vi "子VI-查看某框-不显示界面.vi"(0 "框号":dbl format="%#_13g", 1 "框组":T3(array[cluster]), 2 "计入缺陷的Z值阈值":i32 caption="值", 3 "临界Z值":i32, 4 "计入缺陷的面积阈值":i32, 5 "临界面积百分比值":dbl, 6 "图像Y向分辨率（mm/像素）":dbl, 7 "缺陷灰度阈值":dbl caption="值", 8 "?":T2(plugin-control), 9 "部位信息":string[](array[string])=["", "34.500000", "32.500000", "1121", "34", "54.955926", "分层类", "不合格", ""], 10 "判定为筋条的长宽比阈值":i32, 11 "图像X向分辨率（mm/像素）":dbl) -> (20 "全部检测结果":string[][](table))   [LabVIEW 2018]
uses:
  <vilib>/vision/NI_Vision_Development_Module.lvlib
panel:
  out "中心Y":dbl
  out "中心X":dbl
  in  "Tab Control":T1
  out "Threshold Image":T2(plugin-control)
  out "分层缺陷个数":i32
  out "合格？ 弥散类":string="fencengThreshold"
  out "合格？分层类":string="fencengThreshold"
  out "面积 (pixels)":i32
  in  "格式字符串 2":string="%f"
  in  "分隔符（'\\'代码显示）":string="\t"
  out "分层测量结果":i16[][](array[numeric])
  # "所选区域信息"
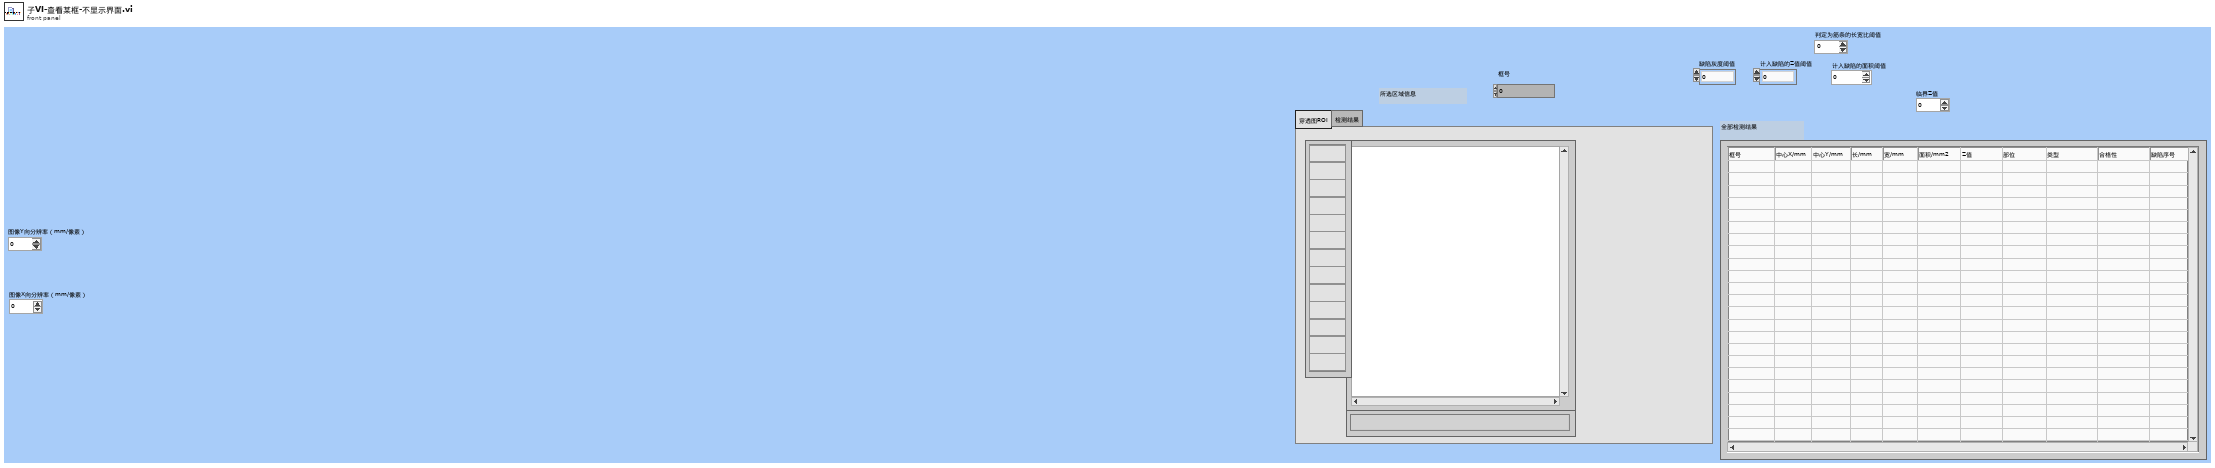
[diagram p1: front panel]
types:
  T1 = typedef "控件2.ctl" = enum32{"穿透图ROI", "检测结果"}
  T2 = typedef "IMAQ Image.ctl" = refnum<image>
  T3 = cluster{"Global Rectangle":i32[], "Contours":cluster{"Contour Type":u32, "ROI Type":u32, "Points":i32[]}[]}[]
  T4 = typedef "Image Type" = u32
  T5 = cluster{"Global Rectangle":i32[], "Contours":cluster{"Contour Type":u32, "ROI Type":u32, "Points":i32[]}[]}
  T6 = cluster{"Desired Font (Application)":enum16{"User-specified Font", "Application Font", "System Font", "Dialog Font"}, "[User-specified Font]":cluster{"Font Name":string, "Size":i16, "Strikeout?":bool, "Italic?":bool, "Underline?":bool, "Outline?":bool, "Shadow?":bool, "Bold?":bool, "Rotation Angle":dbl}, "Horizontal Alignment":i16, "Vertical Alignment":i16}
  T7 = cluster{"histogram":u32[], "Minimal Value":sgl, "Maximal Value":sgl, "Starting Value":sgl, "Interval Width":sgl, "Mean Value":sgl, "Standard  Variation":sgl, "Area (pixels)":i32}
  T8 = typedef "Particle Parameters" = i32
  T9 = cluster{"Area":dbl, "Number of Holes":dbl, "Bounding Rect":cluster{"Left":dbl, "Top":dbl, "Right":dbl, "Bottom":dbl}, "Center of Mass":cluster{"X":dbl, "Y":dbl}, "Orientation":dbl, "Dimensions":cluster{"Width":dbl, "Height":dbl}}[]
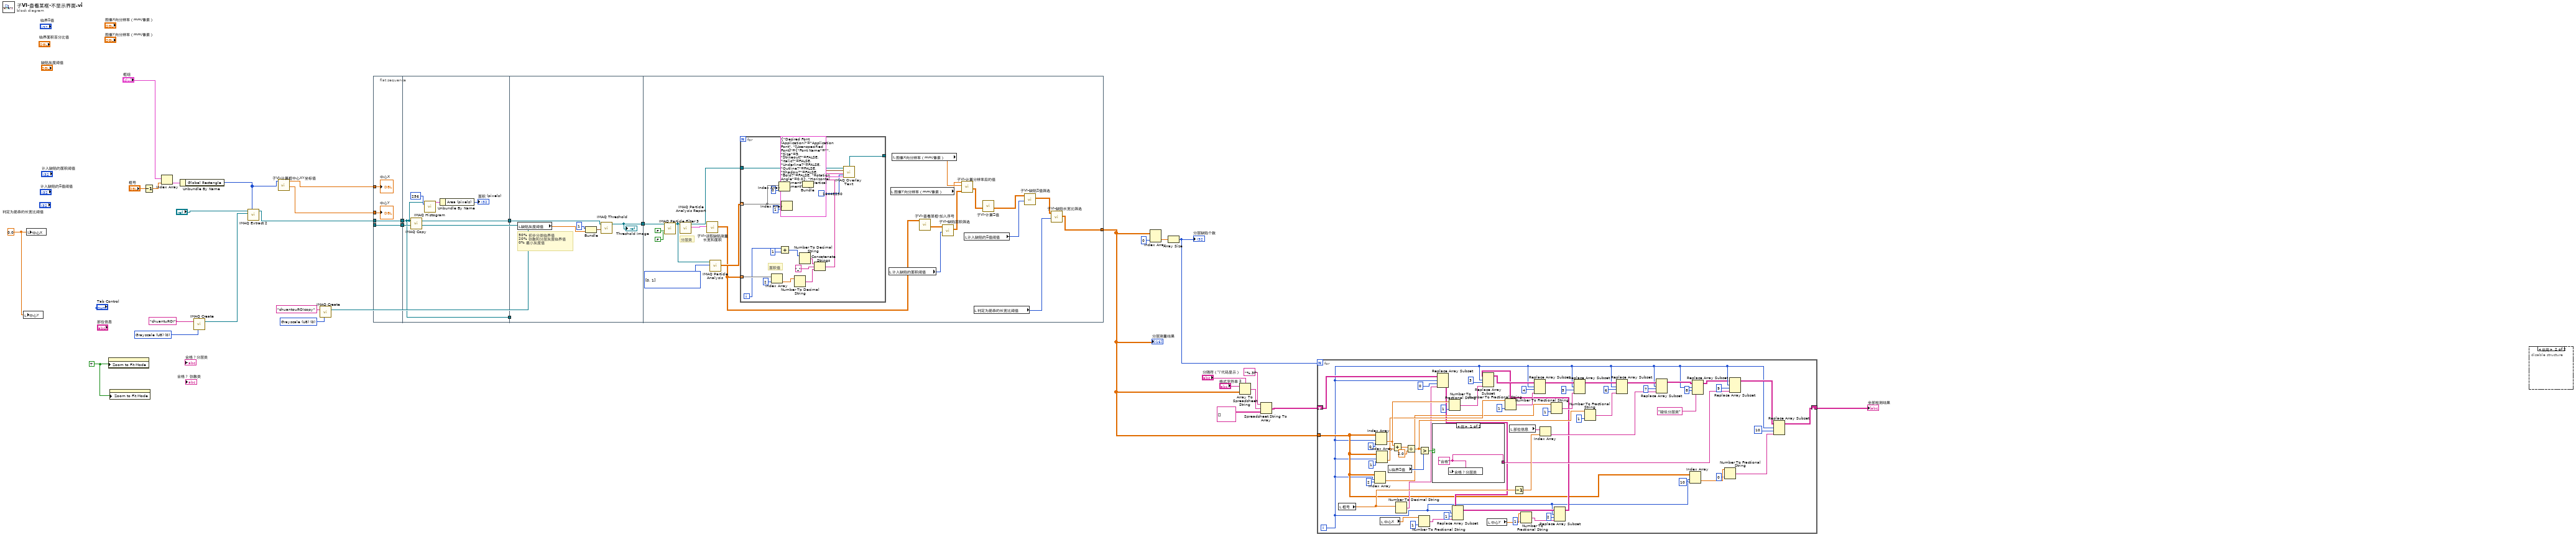
[diagram p0: block diagram]
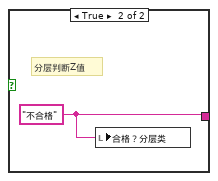
[diagram p2: hidden frame]
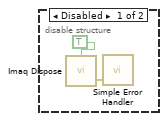
[diagram p3: hidden frame]
diagram:
  w4 = 0.0 ("中心X")
  w8 = T4 0 items=["Grayscale (U8)", "Grayscale (I16)", "Grayscale (SGL)", "Complex (CSG)", "RGB (U32)", "HSL (U32)", "RGB (U64)", "Grayscale (U16)"] ("Image Type")
  w13 = TRUE ("Zoom to Fit Mode")
  w28 = T4 0 items=["Grayscale (U8)", "Grayscale (I16)", "Grayscale (SGL)", "Complex (CSG)", "RGB (U32)", "HSL (U32)", "RGB (U64)", "Grayscale (U16)"] ("Image Type")
  n1 = local write "中心Y"(w4) -> ()
  n2 = local write "中心X"(w4) -> ()
  n3 = property class="ImageControl"("Zoom to Fit Mode"=w13) -> ()  [unwired: 2 in, 2 out]
  n4 = property class="ImageControl"("Zoom to Fit Mode"=w13) -> ()  [unwired: 2 in, 2 out]
  n5 = Decrement(x="框号") -> (x-1=w30:dbl)
  n6 = Index Array(array="框组", index=w30) -> (element=w31:T5)
  n7 = Unbundle By Name(w31) -> ("Global Rectangle"=w7:i32[])
  n8 = call "IMAQ Create"("Image Name"="chuantuROI", "Image Type"=w28) -> ("New Image"=w27:T2)  [unwired: 3 in, 1 out]
  n9 = call "IMAQ Extract 2"("Optional Rectangle"=w7, "Image Dst"=w27, "Image Src"="?") -> ("Image Dst Out"=w1:T2)  [unwired: 7 in, 1 out]
  n10 = call "子VI-计算框中心XY坐标值.vi"("Global Rectangle"=w7) -> ("中心Y"=w5:dbl, "中心X"=w6:dbl)  [unwired: 9 in]
  n11 = call "IMAQ Create"("Image Name"="chuantouROIcopy", "Image Type"=w8) -> ("New Image"=w11:T2)  [unwired: 3 in, 1 out]
  n12 = flat-sequence {
    tunnel: w1 -> [w37]
    tunnel: [w37] -> w14
    tunnel: w11 -> [w36]
    tunnel: [w36] -> w10
    tunnel: w6 -> [w35]
    tunnel: w5 -> [w34]
    tunnel: [w40] -> w15
    tunnel: w14 -> [w40]
    tunnel: [w39] -> w12
    tunnel: w10 -> [w38]
    tunnel: [w48] -> w24
    tunnel: w15 -> [_]
    tunnel: w12 -> [w47]
    tunnel: [w60] -> w17
    tunnel: w24 -> [w66]
    frame #0 {
      "中心X" <- w35
      "中心Y" <- w34
    }
    frame #1 {
      n13 = call "IMAQ Copy"("Image Dst"=w38, "Image Src"=w40) -> ("Image Dst Out"=w39:T2)  [unwired: 4 in, 1 out]
      n14 = call "IMAQ Histogram"("Number of Classes"=256, "Image"=w40) -> ("Histogram Report"=w42:T7)  [unwired: 8 in, 1 out]
      n15 = Unbundle By Name(w42) -> ("Area (pixels)"=→"面积 (pixels)":i32)
    }
    frame #2 {
      # "50% 初步分类临界值\n20% 弥散和分层灰度临界值\n0% 最小灰度值"
      n16 = local read "缺陷灰度阈值"() -> (w45:dbl)
      n17 = Bundle(1, "缺陷灰度阈值"=w45) -> (w44:cluster{i32, "缺陷灰度阈值":dbl})  [unwired: 1 in]
      n18 = call "IMAQ Threshold"("Range"=w44, "Image Src"=w47) -> ("Image Dst Out"=w48:T2)  [unwired: 4 in, 5 out]
      "Threshold Image" <- w48
    }
    frame #3 {
      w54 = T8[] [0, 1] items=["Center of Mass X", "Center of Mass Y", "First Pixel X", "First Pixel Y", "Bounding Rect Left", "Bounding Rect Top", "Bounding Rect Right", "Bounding Rect Bottom", "Max Feret Diameter Start X", "Max Feret Diameter Start Y", "Max Feret Diameter End X", "Max Feret Diameter End Y", "Max Horiz. Segment Length Left", "Max Horiz. Segment Length Right", "Max Horiz. Segment Length Row", "-", "Bounding Rect Width", "Bounding Rect Height", "Bounding Rect Diagonal", "Perimeter", "Convex Hull Perimeter", "Holes' Perimeter", "Max Feret Diameter", "Equivalent Ellipse Major Axis", "Equivalent Ellipse Minor Axis", "Equivalent Ellipse Minor Axis (Feret)", "Equivalent Rect Long Side", "Equivalent Rect Short Side", "Equivalent Rect Diagonal", "Equivalent Rect Short Side (Feret)", "Average Horiz. Segment Length", "Average Vert. Segment Length", "Hydraulic Radius", "Waddel Disk Diameter", "-", "Area", "Holes' Area", "Particle & Holes' Area", "Convex Hull Area", "Image Area", "-", "Number of Holes", "Number of Horiz. Segments", "Number of Vert. Segments", "-", "Orientation", "Max Feret Diameter Orientation", "-", "% Area/Image Area", "% Area/(Particle & Holes' Area)", "Ratio of Equivalent Ellipse Axes", "Ratio of Equivalent Rect Sides", "-", "Elongation Factor", "Compactness Factor", "Heywood Circularity Factor", "Type Factor", "-", "Sum X", "Sum Y", "Sum XX", "Sum XY", "Sum YY", "Sum XXX", "Sum XXY", "Sum XYY", "Sum YYY", "-", "Moment of Inertia XX", "Moment of Inertia XY", "Moment of Inertia YY", "Moment of Inertia XXX", "Moment of Inertia XXY", "Moment of Inertia XYY", "Moment of Inertia YYY", "Norm. Moment of Inertia XX", "Norm. Moment of Inertia XY", "Norm. Moment of Inertia YY", "Norm. Moment of Inertia XXX", "Norm. Moment of Inertia XXY", "Norm. Moment of Inertia XYY", "Norm. Moment of Inertia YYY", "Hu Moment 1", "Hu Moment 2", "Hu Moment 3", "Hu Moment 4", "Hu Moment 5", "Hu Moment 6", "Hu Moment 7"] ("Pixel Measurements")
      # "分层类"
      n19 = call "IMAQ Particle Filter 3"("Image Src"=w66, "Keep/Remove Particles (F)"=FALSE, "Reject Border? (F)"=FALSE) -> ("Image Dst Out"=w53:T2)  [unwired: 10 in, 2 out]
      n20 = call "IMAQ Particle Analysis Report"("Image"=w53) -> ("Particle Reports (Pixels)"=w65:T9, "Image Out (duplicate)"=w51:T2)  [unwired: 5 in, 4 out]
      n21 = call "子VI-读取缺陷测量长宽和面积.vi"("Particle Reports (Pixels)"=w65) -> ("测量结果"=w50:dbl[][])  [unwired: 10 in]
      n22 = call "IMAQ Particle Analysis"("Pixel Measurements"=w54, "Image"=w53) -> ("Particle Measurements (Pixels)"=w52:dbl[][])  [unwired: 4 in, 5 out]
      n23 = for {
        tunnel: [w80] -> _
        tunnel: w51 -> [w88]
        tunnel: w52 -> [w85] mode=indexing
        tunnel: w50 -> [w76] mode=indexing
        i -> [w71]
        # "面积值"
        n24 = Index Array(array=w76, index=2 ("索引")) -> (element=w83:dbl)
        n25 = Index Array(array=w85, index=0 ("索引")) -> (element=w79:dbl)
        n26 = Add(x=w71, y=1) -> (x+y=w69:i32)
        n27 = Index Array(array=w85, index=1 ("索引")) -> (element=w78:dbl)
        n28 = Number To Decimal String(number=w83) -> (decimal integer string=w73:string)  [unwired: 1 in]
        n29 = Number To Decimal String(number=w69) -> (decimal integer string=w75:string)  [unwired: 1 in]
        n30 = Bundle("Numeric"=w79, "Numeric"=w78) -> (w77:cluster{"Numeric":dbl, "Numeric":dbl})  [unwired: 1 in]
        n31 = Concatenate Strings(w75, "_" ("字符串"), w73) -> (w74:string)
        n32 = call "IMAQ Overlay Text"("Text Color (black)"=u32 16448250, "Font, Size & Style"=T6 {"Desired Font (Application)"=enum."Application Font", "[User-specified Font]"={"Font Name"="", "Size"=9, "Strikeout?"=FALSE, "Italic?"=FALSE, "Underline?"=FALSE, "Outline?"=FALSE, "Shadow?"=FALSE, "Bold?"=FALSE, "Rotation Angle"=0.0}, "Horizontal Alignment"=0, "Vertical Alignment"=0}, "String"=w74, "Origin"=w77, "Image"=w88) -> ("Image Out"=w80:T2)  [unwired: 5 in, 1 out]
      }
      n33 = local read "计入缺陷的面积阈值"() -> (w64:i32)
      n34 = local read "图像Y向分辨率（mm/像素）"() -> (w55:dbl)
      n35 = local read "图像X向分辨率（mm/像素）"() -> (w56:dbl)
      n36 = call "子VI-查看某框-加入序号.vi"("测量结果"=w50) -> ("测量结果 3"=w49:dbl[][])  [unwired: 9 in]
      n37 = call "子VI-缺陷面积筛选.vi"("计入分层缺陷的面积阈值"=w64, "分层测量结果"=w49) -> ("初始化的数组"=w58:dbl[][])  [unwired: 8 in, 1 out]
      n38 = call "子VI-计算分辨率后的值.vi"("测量结果"=w58, "图像X向分辨率（mm/像素）"=w56, "图像Y向分辨率（mm/像素）"=w55) -> ("初始化的数组"=w57:dbl[][])  [unwired: 7 in]
      n39 = local read "计入缺陷的Z值阈值"() -> (w63:i32)
      n40 = local read "判定为筋条的长宽比阈值"() -> (w59:i32)
      n41 = call "子VI-计算Z值.vi"("分层测量结果"=w57) -> ("初始化的数组"=w62:dbl[][])  [unwired: 9 in]
      n42 = call "子VI-缺陷Z值筛选.vi"("计入缺陷的Z值阈值"=w63, "分层测量结果"=w62) -> ("初始化的数组"=w61:dbl[][])  [unwired: 8 in, 1 out]
      n43 = call "子VI-缺陷长宽比筛选.vi"("判定为筋条的长宽比阈值"=w59, "分层测量结果"=w61) -> ("初始化的数组"=w60:dbl[][])  [unwired: 9 in]
    }
  }
  n44 = Index Array(array=w17, index (col)=0 ("禁用的索引 (列)")) -> (element=w26:dbl[])  [unwired: 1 in]
  n45 = Array Size(array=w26) -> (size(s)=w23:i32)
  "分层缺陷个数" <- w23
  n46 = Array To Spreadsheet String(delimiter (Tab)="分隔符（'\\'代码显示）", array=w17, 3:"格式字符串 2") -> (spreadsheet string=w20:string)
  n47 = Spreadsheet String To Array(format string="%.3f", spreadsheet string=w20, array type (2D Dbl)=string[][] [] ("Array")) -> (array=w16:string[][])  [unwired: 1 in]
  n48 = for {
    N: w23 -> [_]
    tunnel: w17 -> [w95]
    shift-right: [w99] -> w3
    shift-left: w16 -> [w133]
    i -> [w92]
    n49 = local read "框号"() -> (w140:dbl)
    n50 = Index Array(array=w95, index (row)=w92, index (col)=2 ("索引 (列)")) -> (element=w118:dbl)
    n51 = Index Array(array=w95, index (row)=w92, index (col)=0 ("禁用的索引 (列)")) -> (element=w125:dbl)
    n52 = Index Array(array=w95, index (row)=w92, index (col)=1 ("禁用的索引 (列)")) -> (element=w124:dbl)
    n53 = local read "中心X"() -> (w115:dbl)
    n54 = local read "临界Z值"() -> (w147:i32)
    n55 = Add(x=w125, y=w124) -> (x+y=w148:dbl)
    n56 = Number To Decimal String(number=w140) -> (decimal integer string=w117:string)  [unwired: 1 in]
    n57 = Divide(x=w148, y=2.0) -> (x/y=w122:dbl)
    n58 = Number To Fractional String(number=w115, precision (6)=i16 1 ("精度(6)")) -> (F-format string=w114:string)  [unwired: 2 in]
    n59 = Greater?(x=w122, y=w147) -> (0:w149:bool)
    n60 = case shown="假" w149 {
      tunnel: [w150 w151] -> w120
      frame False {
        w150 = "合格" ("合格？")
        n61 = local write "合格？分层类"(w150) -> ()
      }
      frame True {
        w151 = "不合格" ("合格？")
        # "分层判断Z值"
        n62 = local write "合格？分层类"(w151) -> ()
      }
    }
    n63 = Replace Array Subset(array=w133, new element=w117, index (row)=w92, index (col)=0 ("索引 (列)")) -> (w107:string[][])
    n64 = Number To Fractional String(number=w125, precision (6)=i16 1 ("精度(6)")) -> (F-format string=w132:string)  [unwired: 2 in]
    n65 = Replace Array Subset(array=w107, new element=w114, index (row)=w92, index (col)=1 ("索引 (列)")) -> (w108:string[][])
    n66 = local read "中心Y"() -> (w112:dbl)
    n67 = Number To Fractional String(number=w124, precision (6)=i16 1 ("精度(6)")) -> (F-format string=w131:string)  [unwired: 2 in]
    n68 = local read "部位信息"() -> (w143:string[])
    n69 = Decrement(x=w140) -> (x-1=w142:dbl)
    n70 = Number To Fractional String(number=w112, precision (6)=i16 1 ("精度(6)")) -> (F-format string=w110:string)  [unwired: 2 in]
    n71 = Index Array(array=w143, index=w142) -> (element=w121:string)
    n72 = Number To Fractional String(number=w118, precision (6)=i16 1 ("精度(6)")) -> (F-format string=w128:string)  [unwired: 2 in]
    n73 = Replace Array Subset(array=w108, new element=w110, index (row)=w92, index (col)=2 ("索引 (列)")) -> (w106:string[][])
    n74 = Replace Array Subset(array=w106, new element=w132, index (row)=w92, index (col)=3 ("索引 (列)")) -> (w130:string[][])
    n75 = Replace Array Subset(array=w130, new element=w131, index (row)=w92, index (col)=4 ("索引 (列)")) -> (w129:string[][])
    n76 = Replace Array Subset(array=w129, new element=w128, index (row)=w92, index (col)=5 ("索引 (列)")) -> (w127:string[][])
    n77 = Number To Fractional String(number=w122, precision (6)=i16 1 ("精度(6)")) -> (F-format string=w123:string)  [unwired: 2 in]
    n78 = Replace Array Subset(array=w127, new element=w123, index (row)=w92, index (col)=6 ("索引 (列)")) -> (w126:string[][])
    n79 = Replace Array Subset(array=w126, new element=w121, index (row)=w92, index (col)=7 ("索引 (列)")) -> (w93:string[][])
    n80 = Index Array(array=w95, index (row)=w92, index (col)=10 ("索引 (列)")) -> (element=w97:dbl)
    n81 = Replace Array Subset(array=w93, new element="疑似分层类" ("新元素/子数组"), index (row)=w92, index (col)=8 ("禁用的索引 (列)")) -> (w89:string[][])
    n82 = Number To Fractional String(number=w97, precision (6)=i16 0 ("精度(6)")) -> (F-format string=w94:string)  [unwired: 2 in]
    n83 = Replace Array Subset(array=w89, new element=w120, index (row)=w92, index (col)=9 ("索引 (列)")) -> (w100:string[][])
    n84 = Replace Array Subset(array=w100, new element=w94, index (row)=w92, index (col)=10 ("禁用的索引 (列)")) -> (w99:string[][])
  }
  "全部检测结果" <- w3
  n85 = disable-structure shown="启用" {
    frame Disabled {
      n86 = call "Imaq Dispose"("All Images? (No)"=TRUE) -> ("error out"=w153:errorcluster)  [unwired: 5 in]
      n87 = call <vilib>:"Simple Error Handler.vi"("error in (no error)"=w153) -> ()  [unwired: 4 in, 5 out]
    }
    frame Enabled {
    }
  }
  "分层测量结果" <- w17
